vi "Analyzer.CSVFileNameParser.vi"(8 "error in (no error)":errorcluster, 11 "Requirements Definition (.csv)":path) -> (0 "error out":errorcluster, 2 "No more elements":bool, 3 "Requirements":string[](array[string]))   [LabVIEW 2022 SP3, in "Analyzer.lvclass"]
uses:
  Analyzer.lvclass
  <vilib>/Utility/file.llb/Read Delimited Spreadsheet (string).vi
  Analyzer.lvclass/Analyzer.ctl
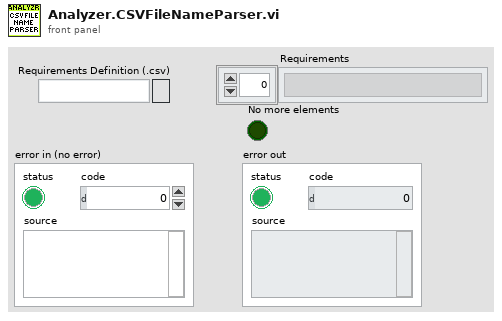
[diagram p1: front panel]
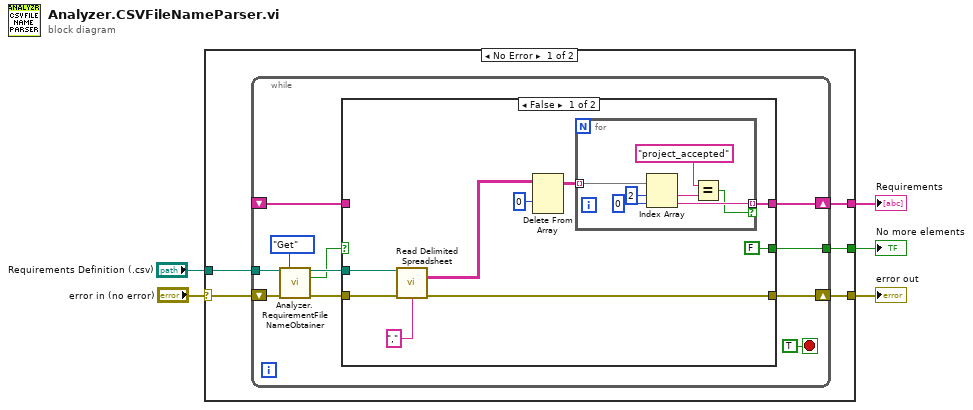
[diagram p0: block diagram]
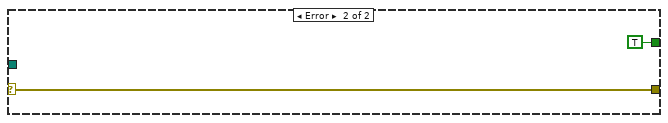
[diagram p3: hidden frame]
diagram:
  n1 = case shown="No Error" "error in (no error)" {
    selector: "error in (no error)" -> [w7 w42]
    tunnel: [w10 w42] -> w5
    tunnel: [w9 _] -> w4
    tunnel: "Requirements Definition (.csv)" -> [w8 _]
    tunnel: [w6 TRUE] -> w1
    frame No Error {
      n2 = while {
        tunnel: w8 -> [w18]
        shift-right: [w20] -> w10
        shift-left: w7 -> [w14]
        shift-right: [w19] -> w9
        shift-left: _ -> [w12]
        tunnel: [w11] -> w6
        stop <- TRUE stop-if-true
        n3 = call "Analyzer.RequirementFileNameObtainer.vi"("CSV Directory"=w18, "Operation"=enum16{"Reset", "Get"}."Get", "error in"=w14) -> ("File Path"=w16:path, "End of List"=w15:bool, "error out"=w17:errorcluster)  [unwired: 10 in]
        n4 = case shown="False" w15 {
          selector: w15 -> [_ w38]
          tunnel: [w28 w40] -> w20
          tunnel: [w25 w39] -> w19
          tunnel: w17 -> [w24 w40]
          tunnel: w16 -> [w23 _]
          tunnel: w12 -> [_ w39]
          tunnel: [FALSE w38] -> w11
          frame False {
            n5 = call-poly <vilib>:"Read Delimited Spreadsheet.vi"("file path (dialog if empty)"=w23, "error in (no error)"=w24, "delimiter (\\t)"="," ("delimiter (\\t)")) -> ("all rows"=w27:string[][], "error out"=w28:errorcluster)  [unwired: 7 in, 4 out]
            n6 = Delete From Array(array=w27, index (row)=0 ("disabled index (col)")) -> (array with subset deleted=w30:string[][])  [unwired: 2 in, 1 out]
            n7 = for {
              tunnel: w30 -> [w31] mode=indexing
              tunnel: [w33] -> w25 mode=indexing if=w32
              n8 = Index Array(array=w31, index #1=2 ("index"), index #2=0 ("index")) -> (element #1=w35:string, element #2=w33:string)
              n9 = Equal?(x="project_accepted" ("y"), y=w35) -> (x = y?=w32:bool)
            }
          }
          frame True {
          }
        }
      }
    }
    frame Error {
    }
  }
  "error out" <- w5
  "Requirements" <- w4
  "No more elements" <- w1
